vi "Error Empty Executable Name.vi"() -> (0 "Invalid Executable Name":errorcluster)   [LabVIEW 2024, in "serenial.io-ase.lvlib" / "ase.lvclass"]
doc: "Error constant"
uses:
  ase.lvclass
  ase.lvclass/ase.ctl
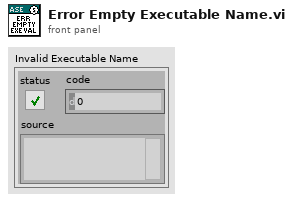
[diagram p1: front panel]
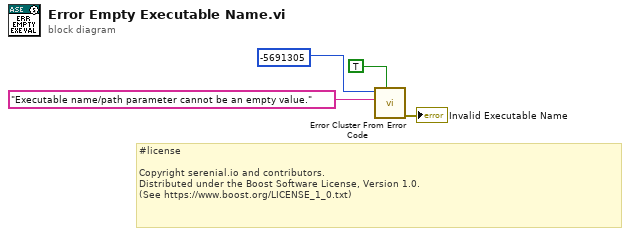
[diagram p0: block diagram]
diagram:
  # "#license\n\nCopyright serenial.io and contributors.\nDistributed under the Boost Software License, Version 1.0.\n(See https://www.boost.org/LICENSE_1_0.txt)"
  n1 = call <vilib>:"Error Cluster From Error Code.vi"("show call chain? (False)"=TRUE, "error message (\"\")"="Executable name/path parameter cannot be an empty value." ("error message (\"\")"), "error code (0)"=-5691305) -> ("error out"=→"Invalid Executable Name":errorcluster)  [unwired: 6 in]
